vi "MDriveCommand.vi"(4 "Channel Name":string, 6 "Port Name":string, 8 "Numeric Value":dbl format="%.2f", 9 "MDriveCommand":T2="DePowerMotor", 10 "Address":i8) -> (0 "String Reply":string, 1 "Error Description":string, 2 "Numeric Reply":dbl, 3 "OK":bool)   [LabVIEW 2016]
uses:
  MDriveDriveCommand.ctl
  CommandDescriptor.ctl
  ~subVIs/CommandPhases.ctl
  ~subVIs/GenericDriveCommand.ctl
panel:
  out "CommandDescriptorOutput":T1
  out "Audit trail":string[](array[string])
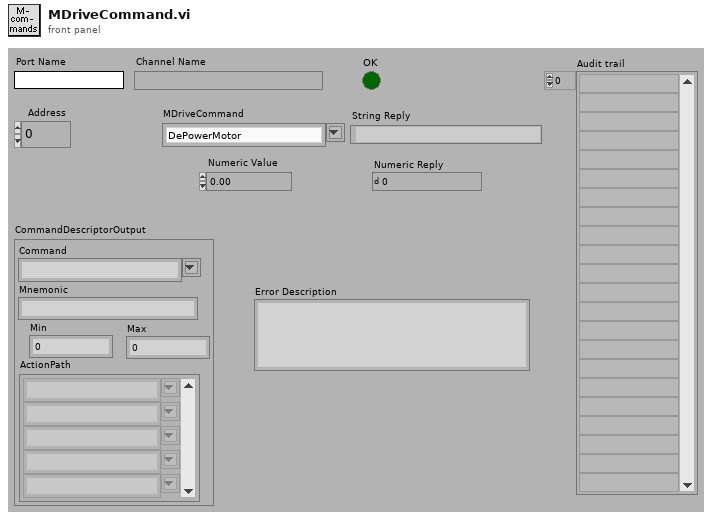
[diagram p1: front panel]
types:
  T1 = typedef "CommandDescriptor.ctl" = cluster{"Command":T2, "Mnemonic":string, "Min":dbl, "Max":dbl, "ActionPath":T3[]}
  T2 = typedef "MDriveDriveCommand.ctl" = string
  T3 = typedef "CommandPhases.ctl" = string
  T4 = typedef "GenericDriveCommand.ctl" = string
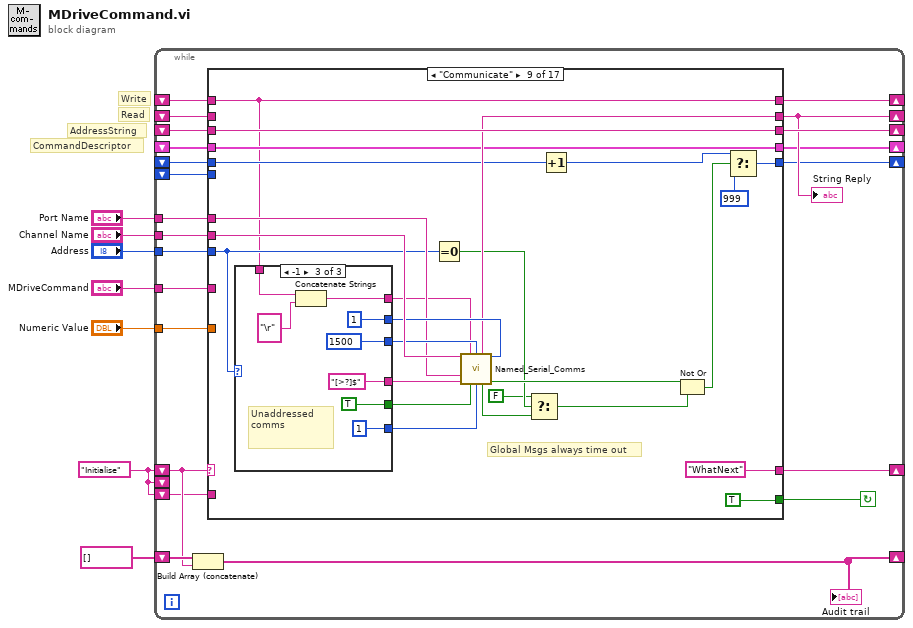
[diagram p0: block diagram]
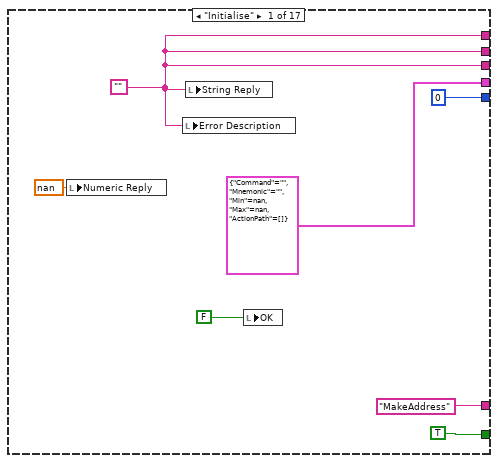
[diagram p2: hidden frame]
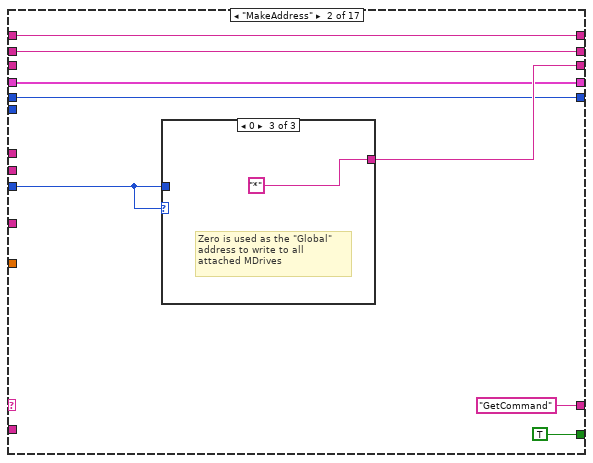
[diagram p3: hidden frame]
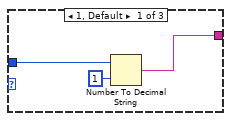
[diagram p4: hidden frame]
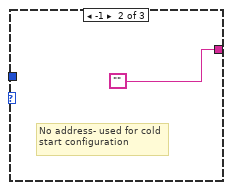
[diagram p5: hidden frame]
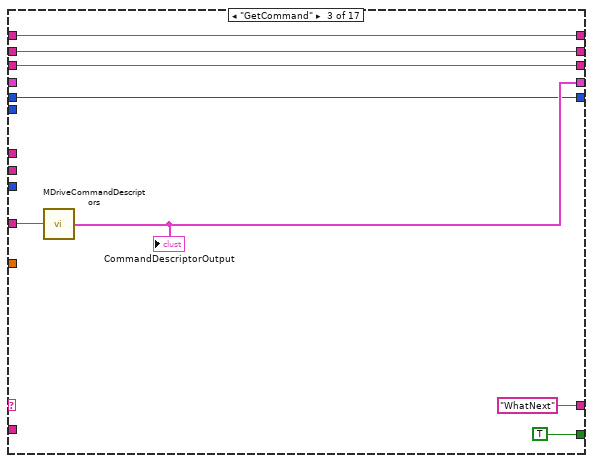
[diagram p6: hidden frame]
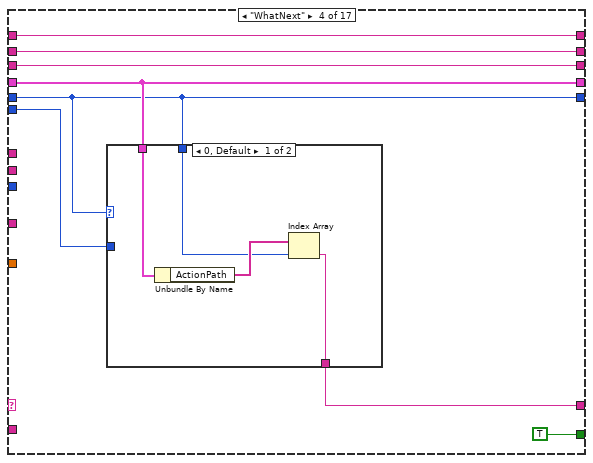
[diagram p7: hidden frame]
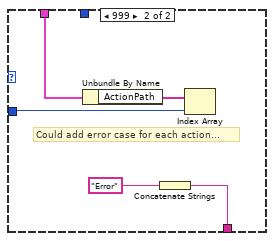
[diagram p8: hidden frame]
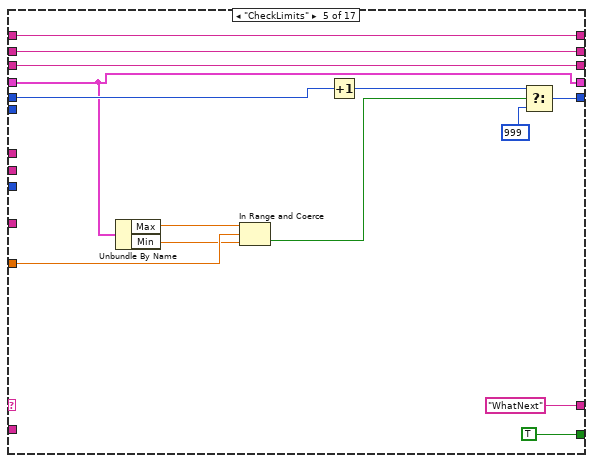
[diagram p9: hidden frame]
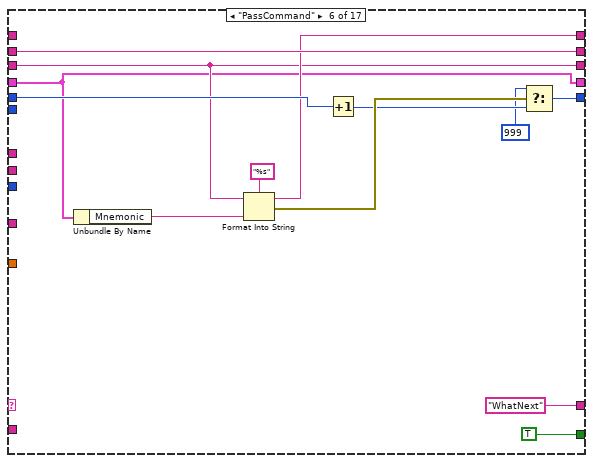
[diagram p10: hidden frame]
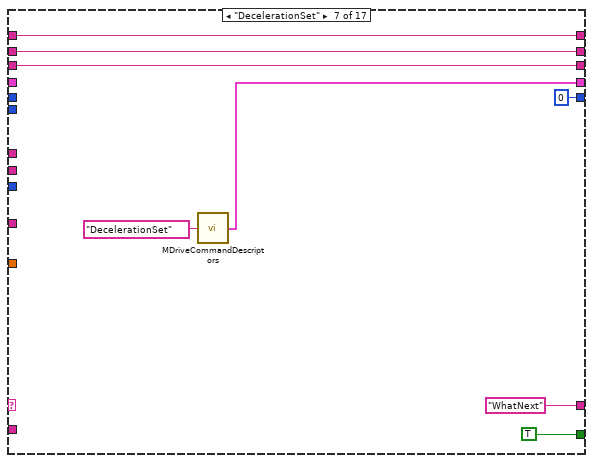
[diagram p11: hidden frame]
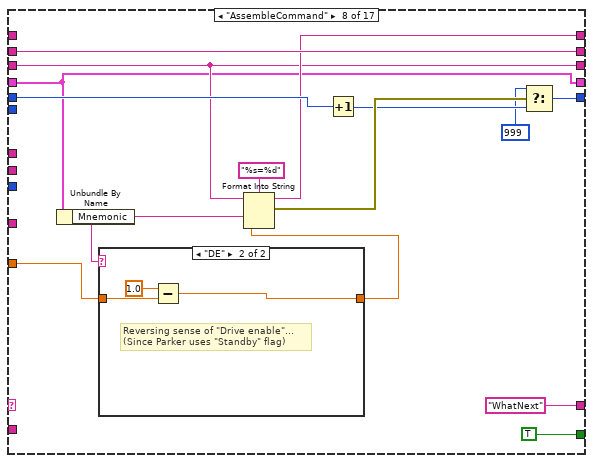
[diagram p12: hidden frame]
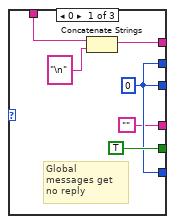
[diagram p14: hidden frame]
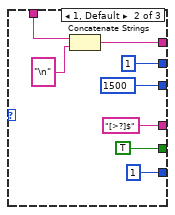
[diagram p15: hidden frame]
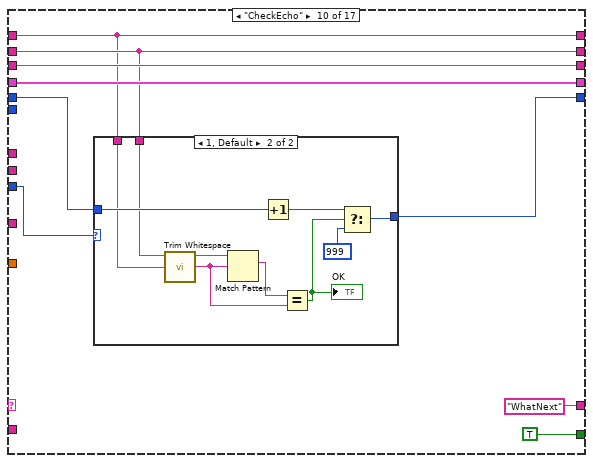
[diagram p16: hidden frame]
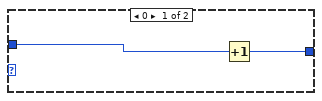
[diagram p17: hidden frame]
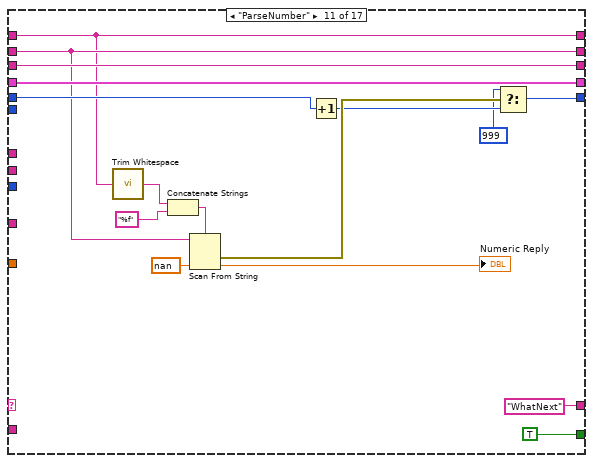
[diagram p18: hidden frame]
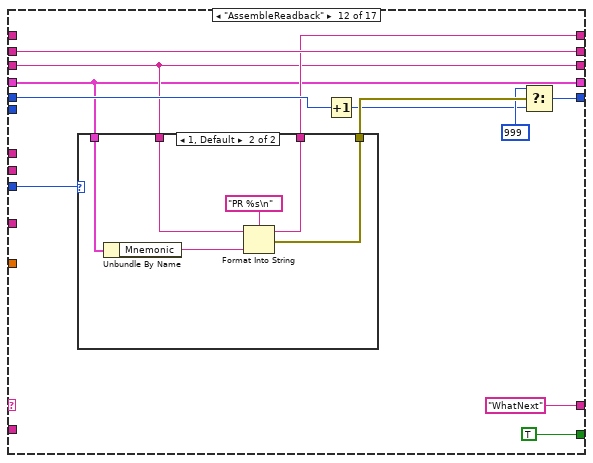
[diagram p19: hidden frame]
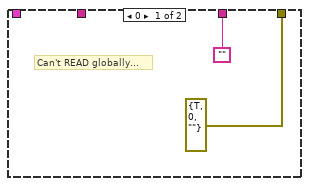
[diagram p20: hidden frame]
diagram:
  w1 = "Initialise"
  # "CommandDescriptor"
  # "AddressString"
  # "Read"
  # "Write"
  n1 = while {
    shift-right: [w17] -> _
    shift-left: w1 -> [w10]
    tunnel: "Address" -> [w29]
    tunnel: "MDriveCommand" -> [w28]
    tunnel: "Numeric Value" -> [w27]
    shift-right: [w26] -> _
    shift-left: _ -> [w25]
    tunnel: "Port Name" -> [w24]
    tunnel: "Channel Name" -> [w23]
    shift-right: [w15] -> _
    shift-left: _ -> [w22]
    shift-right: [w20] -> _
    shift-left: _ -> [w19]
    shift-right: [w16] -> _
    shift-left: string[] [] -> [w18]
    shift-right: [w14] -> _
    shift-left: _ -> [w13]
    shift-right: [w11] -> _
    shift-left: _ -> [w12]
    shift-left: _ -> [w9]
    shift-left: w1 -> [_]
    shift-left: w1 -> [w8]
    stop <- w21 continue-if-true
    n2 = Build Array (concatenate)(w18, w10) -> (w16:T3[])
    "Audit trail" <- w16
    n3 = case shown="\"Communicate\"" w10 {
      selector: w10 -> [_ _ _ _ _ _ _ _ _ _ _ _ _ _ _ _ w305]
      tunnel: ["MakeAddress" "GetCommand" "WhatNext" w61 "WhatNext" "WhatNext" "WhatNext" "WhatNext" "WhatNext" "WhatNext" "WhatNext" "WhatNext" w235 "Error" "Initialise" "Initialise" w305] -> w17
      tunnel: w29 -> [_ w37 _ _ _ _ _ _ w131 w176 _ w215 _ _ _ _ _]
      tunnel: w28 -> [_ _ w54 _ _ _ _ _ _ _ _ _ _ _ _ _ _]
      tunnel: w27 -> [_ _ _ _ w86 _ _ w111 _ _ _ _ _ _ _ w290 _]
      tunnel: [w31 w42 w56 w64 w84 w96 w103 w119 w130 w177 w198 w218 w241 w257 w285 w296 w303] -> w26
      tunnel: w25 -> [_ w42 w56 w64 w84 _ w103 _ w130 w177 w198 _ w241 w257 w278 _ _]
      tunnel: w24 -> [_ _ _ _ _ _ _ _ w147 _ _ _ _ _ w279 _ _]
      tunnel: w23 -> [_ _ _ _ _ _ _ _ w153 _ _ _ _ w252 w280 _ _]
      tunnel: [w31 w41 w55 w63 w88 w101 w109 w124 w144 w178 w205 w223 w239 w262 w285 w296 w303] -> w15
      tunnel: w22 -> [_ w41 w55 w63 w88 w101 w109 w124 _ w178 w205 w223 w239 w262 w277 _ _]
      tunnel: [TRUE TRUE ("Continue") TRUE ("Continue") TRUE ("Continue") TRUE TRUE TRUE TRUE TRUE TRUE TRUE TRUE w236 TRUE FALSE ("Continue") FALSE ("Continue") FALSE] -> w21
      tunnel: [w31 w44 w53 w62 w87 w95 w106 w118 w145 w183 w210 w216 w240 w267 w285 w296 w303] -> w20
      tunnel: w19 -> [_ _ w53 w62 w87 w95 w106 w118 w145 w183 w210 w216 w240 w267 _ w288 _]
      tunnel: [T1 {"Command"="", "Mnemonic"="", "Min"=nan, "Max"=nan, "ActionPath"=[]} ("CommandDescriptorOutput") w39 w51 w60 w75 w92 w105 w116 w143 w179 w206 w214 w233 w263 w284 w294 w302] -> w14
      tunnel: w13 -> [_ w39 _ w60 w75 w92 _ w116 w143 w179 w206 w214 w232 w263 w284 w294 w302]
      tunnel: w12 -> [_ w38 w50 w59 w79 w97 _ w120 w138 w180 w207 w219 _ w264 w283 w295 w301]
      tunnel: [0 w38 w50 w59 w80 w98 0 ("f") w121 w140 w181 w208 w220 0 ("f") w265 w283 w295 w301] -> w11
      tunnel: w9 -> [_ _ _ w58 _ _ _ _ _ _ _ _ _ _ _ _ _]
      tunnel: w8 -> [_ _ _ _ _ _ _ _ _ _ _ _ _ _ w275 _ _]
      frame "Initialise" {
        w31 = ""
        n4 = local write "Numeric Reply"(nan ("Numeric Reply")) -> ()
        n5 = local write "Error Description"(w31) -> ()
        n6 = local write "String Reply"(w31) -> ()
        n7 = local write "OK"(FALSE ("GoodEcho")) -> ()
      }
      frame "MakeAddress" {
        n8 = case shown="0" w37 {
          tunnel: w37 -> [w46 _ _]
          tunnel: [w45 "" "*"] -> w44
          frame 1, Default {
            n9 = Number To Decimal String(number=w46, width (-)=i16 1) -> (decimal integer string=w45:string)
          }
          frame -1 {
            # "No address- used for cold start configuration"
          }
          frame 0 {
            # "Zero is used as the \"Global\" address to write to all attached MDrives"
          }
        }
      }
      frame "GetCommand" {
        n10 = call "MDriveCommandDescriptors.vi"("MDriveCommand"=w54) -> ("CommandDescriptorOutput"=w51:T1)  [unwired: 4 out]
        "CommandDescriptorOutput" <- w51
      }
      frame "WhatNext" {
        n11 = case shown="0, Default" w59 {
          tunnel: [w68 w71] -> w61
          tunnel: w60 -> [w67 w72]
          tunnel: w59 -> [w66 _]
          tunnel: w58 -> [_ w73]
          frame 0, Default {
            n12 = Unbundle By Name(w67) -> ("ActionPath"=w69:T3[])
            n13 = Index Array(array=w69, index=w66) -> (element=w68:T3)
          }
          frame 999 {
            # "Could add error case for each action..."
            n14 = Unbundle By Name(w72) -> ("ActionPath"=w74:T3[])
            n15 = Concatenate Strings("Error") -> (w71:string)
            n16 = Index Array(array=w74, index=w73) -> ()  [unwired: 1 out]
          }
        }
      }
      frame "CheckLimits" {
        n17 = Unbundle By Name(w75) -> ("Max"=w83:dbl, "Min"=w82:dbl)
        n18 = In Range and Coerce(upper limit=w83, x=w86, lower limit=w82) -> (In Range?=w77:bool)  [unwired: 1 out]
        n19 = Increment(x=w79) -> (x+1=w78:i32)
        n20 = Select(t=w78, s=w77, f=999) -> (s? t:f=w80:i32)
      }
      frame "PassCommand" {
        n21 = Unbundle By Name(w92) -> ("Mnemonic"=w94:string)
        n22 = Format Into String(format string="%s", initial string=w95, w94) -> (resulting string=w96:string, error out=w91:errorcluster)  [unwired: 1 in]
        n23 = Increment(x=w97) -> (x+1=w90:i32)
        n24 = Select(t=999 ("f"), s=w91, f=w90) -> (s? t:f=w98:i32)
      }
      frame "DecelerationSet" {
        n25 = call "MDriveCommandDescriptors.vi"("MDriveCommand"=T4 "DecelerationSet" ("GenericDriveCommand")) -> ("CommandDescriptorOutput"=w105:T1)  [unwired: 4 out]
      }
      frame "AssembleCommand" {
        n26 = Unbundle By Name(w116) -> ("Mnemonic"=w112:string)
        n27 = case shown="\"DE\"" w112 {
          tunnel: w111 -> [w125 w128]
          tunnel: [w125 w126] -> w110
          frame "False", Default {
          }
          frame "DE" {
            # "Reversing sense of \"Drive enable\"...\n(Since Parker uses \"Standby\" flag)"
            n28 = Subtract(x=1.0, y=w128) -> (x-y=w126:dbl)
          }
        }
        n29 = Format Into String(format string="%s=%d", initial string=w118, w112, w110) -> (resulting string=w119:string, error out=w115:errorcluster)  [unwired: 1 in]
        n30 = Increment(x=w120) -> (x+1=w114:i32)
        n31 = Select(t=999 ("f"), s=w115, f=w114) -> (s? t:f=w121:i32)
      }
      frame "Communicate" {
        # "Global Msgs always time out"
        n32 = case shown="-1" w131 {
          tunnel: ["" "[>?]$" "[>?]$"] -> w152
          tunnel: [w158 1 ("Terminate Count") 1 ("Terminate Count")] -> w151
          tunnel: [w158 u32 1500 ("Timeout/ms") u32 1500 ("Timeout/ms")] -> w150
          tunnel: [TRUE ("Log Errors?") TRUE ("Log Errors?") TRUE ("Log Errors?")] -> w149
          tunnel: [w158 1 ("!Error retries") 1 ("!Error retries")] -> w148
          tunnel: w130 -> [w154 w162 w170]
          tunnel: [w155 w161 w169] -> w129
          frame 0 {
            w158 = 0 ("!Error retries")
            # "Global messages get no reply"
            n33 = Concatenate Strings(w154, "\n" ("string")) -> (w155:string)
          }
          frame 1, Default {
            n34 = Concatenate Strings(w162, "\n" ("string")) -> (w161:string)
          }
          frame -1 {
            # "Unaddressed comms"
            n35 = Concatenate Strings(w170, "\r" ("string")) -> (w169:string)
          }
        }
        n36 = Equal To 0?(x=w131) -> (x = 0?=w134:bool)
        n37 = call "Named_Serial_Comms.vi"("Channel Name"=w153, "Write"=w129, "Timeout/ms"=w150, "!Error retries"=w148, "Port Name"=w147, "Term Grep"=w152, "Log Errors?"=w149, "Terminate Count"=w151) -> ("Read"=w144:string, "Timed out"=w133:bool, "Serial Error"=w141:bool)  [unwired: 1 in, 4 out]
        n38 = Select(t=FALSE, s=w134, f=w133) -> (s? t:f=w135:bool)
        n39 = Increment(x=w138) -> (x+1=w137:i32)
        n40 = Not Or(1:w135, 2:w141) -> (0:w139:bool)
        n41 = Select(t=w137, s=w139, f=999) -> (s? t:f=w140:i32)
      }
      frame "CheckEcho" {
        n42 = case shown="1, Default" w176 {
          tunnel: [w185 w194] -> w181
          tunnel: w180 -> [w186 w191]
          tunnel: w178 -> [_ w189]
          tunnel: w177 -> [_ w188]
          frame 0 {
            n43 = Increment(x=w186) -> (x+1=w185:i32)
          }
          frame 1, Default {
            n44 = call <vilib>:"Trim Whitespace.vi"("string"=w188) -> ("trimmed string"=w187:string)  [unwired: 1 in]
            n45 = Match Pattern(string=w189, regular expression=w187) -> (match substring=w190:string)  [unwired: 4 out]
            n46 = Increment(x=w191) -> (x+1=w192:i32)
            n47 = Equal?(x=w190, y=w187) -> (x = y?=w193:bool)
            "OK" <- w193
            n48 = Select(t=w192, s=w193, f=999) -> (s? t:f=w194:i32)
          }
        }
      }
      frame "ParseNumber" {
        n49 = call <vilib>:"Trim Whitespace.vi"("string"=w198) -> ("trimmed string"=w196:string)  [unwired: 1 in]
        n50 = Concatenate Strings(w196, "%f" ("format string")) -> (w199:string)
        n51 = Scan From String(format string=w199, input string=w205, default 1=nan ("default value 1")) -> (error out=w203:errorcluster, output 1=→"Numeric Reply":dbl)  [unwired: 2 in, 2 out]
        n52 = Increment(x=w207) -> (x+1=w202:i32)
        n53 = Select(t=999, s=w203, f=w202) -> (s? t:f=w208:i32)
      }
      frame "AssembleReadback" {
        n54 = case shown="1, Default" w215 {
          tunnel: w214 -> [_ w231]
          tunnel: ["" w230] -> w218
          tunnel: [errorcluster {"status"=TRUE, "code"=0, "source"=""} ("error IO") w229] -> w217
          tunnel: w216 -> [_ w228]
          frame 0 {
            # "Can't READ globally..."
          }
          frame 1, Default {
            n55 = Unbundle By Name(w231) -> ("Mnemonic"=w227:string)
            n56 = Format Into String(format string="PR %s\n", initial string=w228, w227) -> (resulting string=w230:string, error out=w229:errorcluster)  [unwired: 1 in]
          }
        }
        n57 = Increment(x=w219) -> (x+1=w212:i32)
        n58 = Select(t=999 ("f"), s=w217, f=w212) -> (s? t:f=w220:i32)
      }
      frame "Done" {
        n59 = Match Pattern(string=w239, regular expression="?") -> (offset past match=w234:i32)  [unwired: 4 out]
        n60 = case shown="0, Default" w234 {
          tunnel: [TRUE ("Continue") FALSE ("Continue")] -> w236
          tunnel: ["WhatNext" "Initialise"] -> w235
          tunnel: [w244 w246] -> w233
          tunnel: w232 -> [_ w246]
          frame 0, Default {
            n61 = call "MDriveCommandDescriptors.vi"("MDriveCommand"=T4 "GetError" ("GenericDriveCommand")) -> ("CommandDescriptorOutput"=w244:T1)  [unwired: 4 out]
          }
          frame -1 {
          }
        }
      }
      frame "ParseError" {
        n62 = call <vilib>:"Trim Whitespace.vi"("string"=w257) -> ("trimmed string"=w255:string)  [unwired: 1 in]
        n63 = Concatenate Strings(w255, "%s" ("format string")) -> (w258:string)
        n64 = Scan From String(format string=w258, input string=w262, default 1="") -> (error out=w261:errorcluster, output 1=w253:string)  [unwired: 2 in, 2 out]
        n65 = call "MDriveErrorCodes.vi"("Error Code"=w253) -> ("Error Description"=w251:string)  [unwired: 4 out]
        n66 = Increment(x=w264) -> (x+1=w260:i32)
        n67 = Format Into String(format string="The %s has %s", w252, w251) -> (resulting string=→"Error Description":string)  [unwired: 2 in, 1 out]
        n68 = Select(t=999, s=w261, f=w260) -> (s? t:f=w265:i32)
      }
      frame "Error" {
        w272 = "Error in MDriveCommand.vi: " ("string")
        w285 = ""
        n69 = local read "Error Description"() -> (w271:string)
        n70 = call "Serial_log_build.vi"("Read"=w277, "Write String"=w278, "Port Name"=w279) -> ("Output Array"=w281:string[])
        n71 = Empty String/Path?(string/path=w271) -> (empty?=w276:bool)
        n72 = Concatenate Strings(w272, w275) -> (w274:string)
        n73 = Concatenate Strings(w272, w271) -> (w273:string)
        n74 = Select(t=w274, s=w276, f=w273) -> (s? t:f=w270:string)
        n75 = call "Write_serial_log.vi"("Log Type"="MDrive_Error_Log", "Log Array"=w281, "Header message"=w270, "Channel Name"=w280) -> ()  [unwired: 1 out]
        n76 = local write "OK"(FALSE ("GoodEcho")) -> ()
      }
      frame "CheckLimitsError" {
        w296 = ""
        n77 = Unbundle By Name(w294) -> ("Mnemonic"=w291:string)
        n78 = Format Into String(format string="%s=%d) to drive %s", initial string="Attempt to Write an out-of-range value (" ("message"), w291, w290, w288) -> (resulting string=w293:string)  [unwired: 1 in, 1 out]
        n79 = One Button Dialog(message=w293, button name ("OK")="I'll fix it") -> (true=w299:bool)
        n80 = Stop(stop? (T)=w299) -> ()
      }
      frame "NoMatch", Default {
        w303 = ""
        n81 = One Button Dialog(message="Case not found in MDriveCommands.vi", button name ("OK")="Oh Bugger...") -> ()  [unwired: 1 out]
      }
    }
    "String Reply" <- w15
  }
